vi "Hide All Iteration Terminals.vi"(8 "error in (no error)":errorcluster, 11 "VI Ref":refnum<vi>) -> (0 "error out":errorcluster, 2 "Save?":bool, 3 "VI Ref out":refnum<vi>)   [LabVIEW 2020, in "Code Cleanup.lvlib"]
uses:
  Code Cleanup.lvlib
  <vilib>/Utility/traverseref.llb/VI Scripting - Traverse.lvlib
  <vilib>/Utility/traverseref.llb/TRef TravTarget.ctl
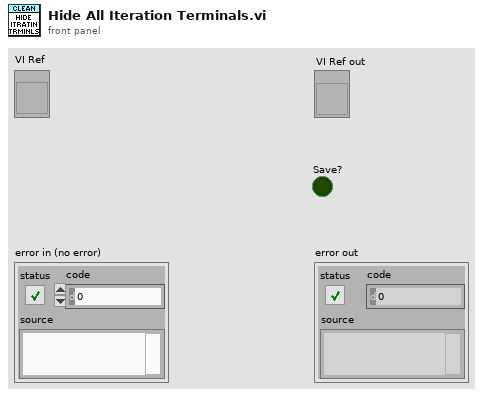
[diagram p1: front panel]
types:
  T1 = typedef "TRef TravTarget.ctl" = enum16{"FP", "BD", "Other"}
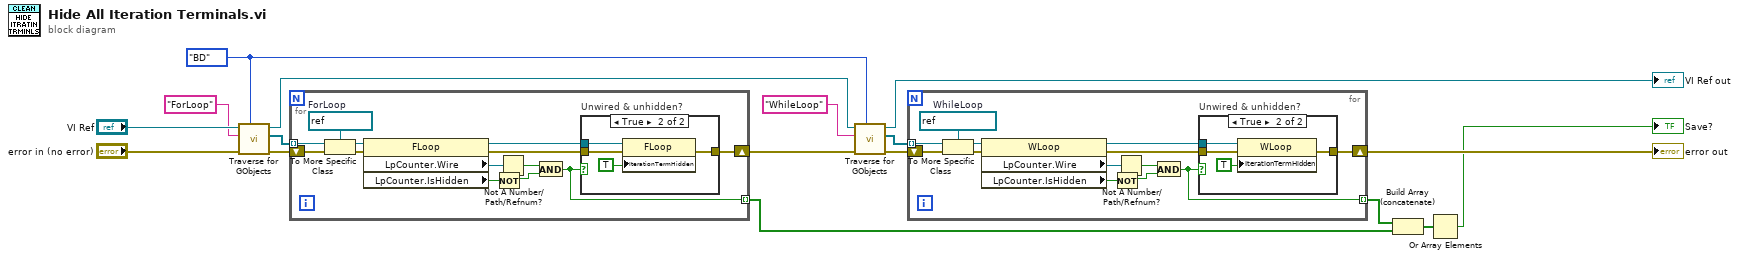
[diagram p0: block diagram]
diagram:
  w13 = TRef_TravTarget."BD" ("Traverse Target")
  n1 = call <vilib>:"Traverse for GObjects.vi"("Traverse Target"=w13, "error in (no error)"="error in (no error)", "Class Name"="ForLoop", "VI Refnum"="VI Ref") -> ("error out"=w15:errorcluster, "References"=w17:refnum<vi>[], "dup VI Refnum"=w16:refnum<vi>)  [unwired: 4 in, 1 out]
  n2 = for {
    tunnel: w17 -> [w30] mode=indexing
    shift-right: [w22] -> w9
    shift-left: w15 -> [w25]
    tunnel: [w18] -> w4 mode=indexing
    w29 = refnum<vi> refnum  # ForLoop
    n3 = To More Specific Class(target class=w29, reference=w30, error in=w25) -> (specific class reference=w28:refnum<vi>, error out=w24:errorcluster)
    n4 = property class="FLoop"(reference=w28, error in=w24) -> (reference out=w27:refnum<vi>, error out=w23:errorcluster, "LpCounter.Wire"=w26:refnum<vi>, "LpCounter.IsHidden"=w21:bool)
    n5 = Not(x=w21) -> (.not. x?=w19:bool)
    n6 = Not A Number/Path/Refnum?(number/path/refnum=w26) -> (NaN/Path/Refnum?=w20:bool)
    n7 = And(x=w20, y=w19) -> (x .and. y?=w18:bool)
    n8 = case "Unwired & unhidden?" shown="True" w18 {
      tunnel: w27 -> [_ w34]
      tunnel: w23 -> [w31 w33]
      tunnel: [w31 w32] -> w22
      frame False {
      }
      frame True {
        n9 = property class="FLoop"(reference=w34, error in=w33, "IterationTermHidden"=TRUE ("Iteration Terminal Hidden?")) -> (error out=w32:errorcluster)  [unwired: 1 out]
      }
    }
  }
  n10 = call <vilib>:"Traverse for GObjects.vi"("Traverse Target"=w13, "error in (no error)"=w9, "Class Name"="WhileLoop", "VI Refnum"=w16) -> ("error out"=w8:errorcluster, "References"=w6:refnum<vi>[], "dup VI Refnum"=→"VI Ref out":refnum<vi>)  [unwired: 4 in, 1 out]
  n11 = for {
    shift-right: [w41] -> w7
    shift-left: w8 -> [w44]
    tunnel: [w37] -> w3 mode=indexing
    tunnel: w6 -> [w36] mode=indexing
    w48 = refnum<vi> refnum  # WhileLoop
    n12 = To More Specific Class(target class=w48, reference=w36, error in=w44) -> (specific class reference=w47:refnum<vi>, error out=w43:errorcluster)
    n13 = property class="WLoop"(reference=w47, error in=w43) -> (reference out=w46:refnum<vi>, error out=w42:errorcluster, "LpCounter.Wire"=w45:refnum<vi>, "LpCounter.IsHidden"=w40:bool)
    n14 = Not(x=w40) -> (.not. x?=w38:bool)
    n15 = Not A Number/Path/Refnum?(number/path/refnum=w45) -> (NaN/Path/Refnum?=w39:bool)
    n16 = And(x=w39, y=w38) -> (x .and. y?=w37:bool)
    n17 = case "Unwired & unhidden?" shown="True" w37 {
      tunnel: w46 -> [_ w52]
      tunnel: w42 -> [w49 w51]
      tunnel: [w49 w50] -> w41
      frame False {
      }
      frame True {
        n18 = property class="WLoop"(reference=w52, error in=w51, "IterationTermHidden"=TRUE ("Iteration Terminal Hidden?")) -> (error out=w50:errorcluster)  [unwired: 1 out]
      }
    }
  }
  "error out" <- w7
  n19 = Build Array (concatenate)(w3, w4) -> (w2:bool[])
  n20 = Or Array Elements(Boolean array=w2) -> (logical OR=→"Save?":bool)
